vi "bbauv_acoustic_sbRIO_v3.vi"() -> ()   [LabVIEW 2012]
doc: "This VI will initialize the FPGA VI and read a user-defined number of samples from a DMA FIFO. When the data acquisition is complete this VI will read status information from the FPGA VI.\n\nFollow these instructions to run the VI.\n\n1. Select your RIO device from the dropdown.\n2. Set the sample period, number of samples to acquire per channel, and DMA block read size. \n\nNote: the block read size should be set to balance load on the host processor and the update rate of the user interface. A small block read size will update the user interface more often but will result in a higher load on the host processor."
uses:
  <vilib>/userdefined/High Color/nirio_resource_hc.ctl
  <vilib>/Analysis/3filter.llb/Filter Passband Type.ctl
  <vilib>/FPGAPlugInAG/sbRIO-9612/niLvFpga_Open_sbRIO-9612.vi
  <vilib>/rvi/interface/common/dynamic/niFpgaDynamicAddResources.vi
  <vilib>/Utility/error.llb/Error Cluster From Error Code.vi
  <vilib>/FPGAPlugInAG/Dynamic/niLvFpga_Run_Dynamic.vi
  <vilib>/rvi/errors/niLvFpgaAdjustHostInterfaceError.vi
  <vilib>/RVI Host/nirviSupport.llb/nirviErrorClusterFromErrorCode.vi
  <vilib>/FPGAPlugInAG/Dynamic/niLvFpga_Close_Dynamic.vi
  <vilib>/Analysis/3filter.llb/Elliptic Filter (DBL).vi
  <vilib>/Analysis/3filter.llb/Butterworth Filter (DBL).vi
  <vilib>/rvi/interface/nirviOpenFPGA/nirviOpenFPGA.xnode
  FPGA Bitfiles/bbauvFPGA_FPGATarget2_NI9223User-Contr_AXBjtBmtN8Y.lvbitx
  NI 9223 User-Controlled IO Sampling (FPGA).vi
  <vilib>/rvi/interface/nirviMethod/nirviMethod.xnode
  <vilib>/rvi/interface/nirviReadWriteControl/nirviReadWriteControl.xnode
  <vilib>/rvi/interface/nirviCloseFPGA/nirviCloseFPGA.xnode
  <vilib>/rvi/errors/niLvFpgaMergeErrorWithErrorCode.vi
  <vilib>/rvi/interface/Simulation/niFpgaSimulationCallBeginRW.vi
  <vilib>/FPGAPlugInAG/Dynamic/niLvFpga_ReadFifo_Dynamic.vi
  <vilib>/rvi/interface/nirviMethod/StockFPGA_InlinedMethodWaitForSingleIRQ.vi
  <vilib>/FPGAPlugInAG/Dynamic/niLvFpga_WaitOnIrq_Dynamic.vi
  <vilib>/FPGAPlugInAG/Dynamic/niLvFpga_AcknowledgeIrq_Dynamic.vi
  NiFpgaLv.dll
  <vilib>/FPGAPlugInAG/Dynamic/niLvFpga_ConfigureFifo_Dynamic.vi
  <vilib>/FPGAPlugInAG/Dynamic/niLvFpga_StartFifo_Dynamic.vi
  <vilib>/Analysis/NI_AALBase.lvlib
panel:
  out "Frequency":dbl
  in  "Noise length":i32=300
  out "Index 0":dbl
  out "Index 1":dbl
  out "Index 2":dbl
  out "Index 3":dbl
  out "amplitude 0":dbl
  out "amplitude 1":dbl
  out "amplitude 2":dbl
  out "amplitude 3":dbl
  in  "Portion Duration":i32=1000
  out "Threshold 0":dbl
  out "Threshold 1":dbl
  out "Threshold 2":dbl
  out "Threshold 3":dbl
  in  "threshold ratio":dbl=3.0
  in  "Display":bool
  in  "Filter mode":enum16{"Elliptic", "Butterworth"}(ring)=enum."Butterworth"
  out "Selected Index":i32
  out "Ratio at Index (%)":dbl
  in  "Threshold":dbl=0.3
  in  "Order":i32=3
  in  "Low Cutoff":dbl=20000.0
  in  "High Cutoff":dbl=26000.0
  in  "Selection:":dbl=25000.0
  out "Freq 2":dbl
  out "Freq 1":dbl
  out "Original Filtered Ch0":dbl[](graph)
  out "bad signal?":bool
  out "dt1":dbl
  out "dt2":dbl
  out "dt3":dbl
  out "ROS  Error":bool
  in  "Send to ROS":bool=TRUE
  in  "Altitude":dbl=2.0
  out "x":dbl format="%#_6f"
  out "y":dbl format="%#_6f"
  out "z":dbl
  out "yaw":dbl
  out "pitch":dbl
  in  "Mode":T1(ring)=enum."Use Far Field"
  out "Forward":dbl
  out "Sidemove":dbl
  out "Arrival Analysis Signal":dbl[][](graph)
  out "Yaw Chart":dbl(graph)
  out "noise index":dbl[](array[numeric])
  out "Frequency Selected Signal":dbl[](graph)
  out "#Elements Acquired":u32(graph)
  in  "Sampling Duration (us)":u32=2005000
  in  "RIO Device":T2="RIO0"
  out "Timed Out":bool
  out "Sample Gated":bool
  out "Overwrite":bool
  in  "Acquisition Stop":bool
  # "Signal Acquisition Control"
  # "TDOA Analysis"
  # "Arrival Analysis"
  # "Frequency Analysis"
  # "TDOA Result"
  # "ROS Communication"
  # "Frequency Analysis"
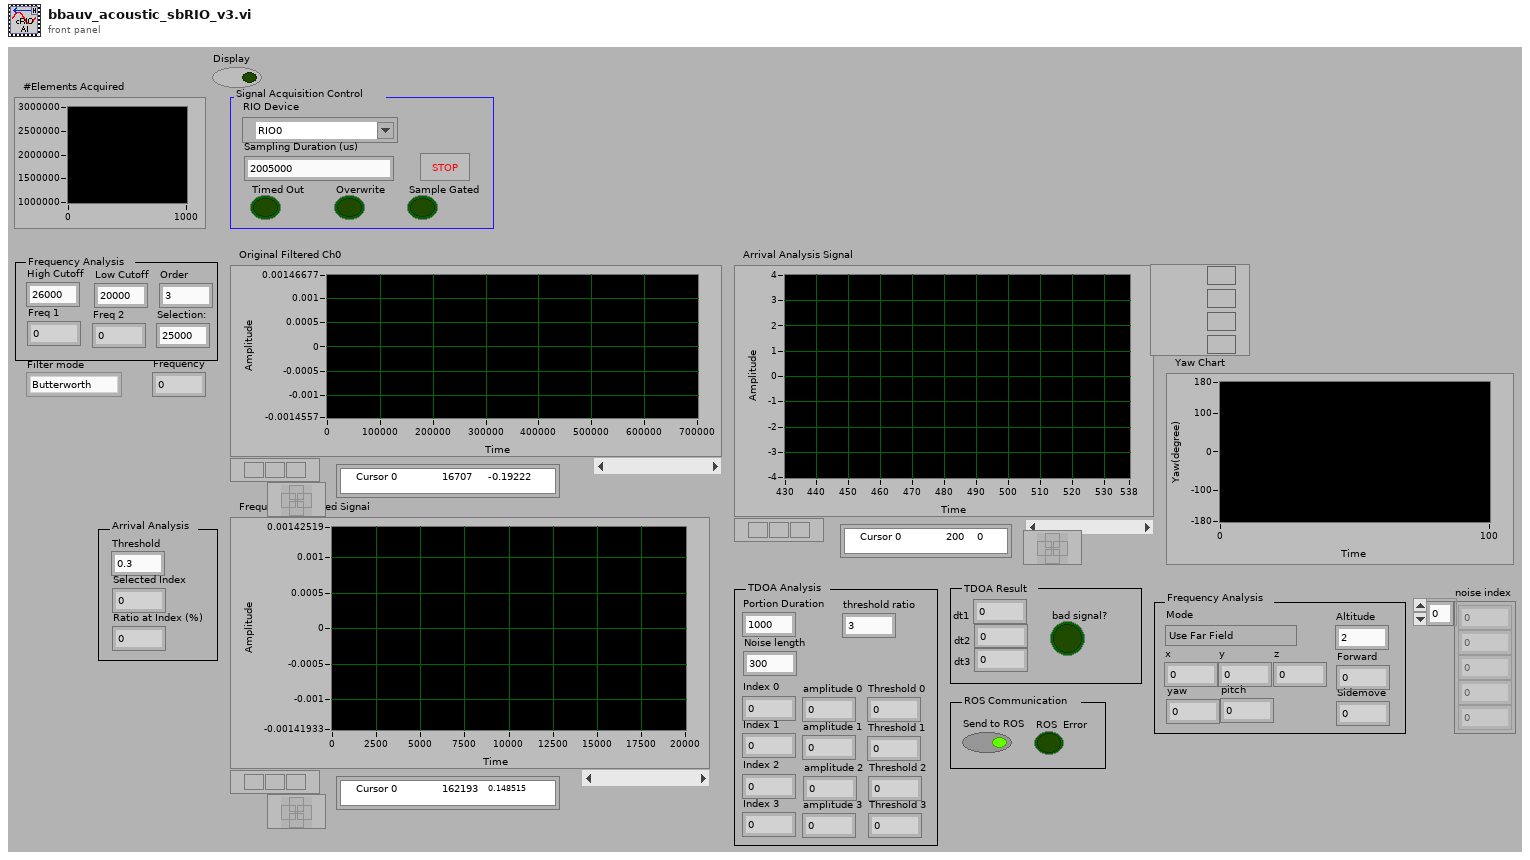
[diagram p1: front panel]
types:
  T1 = enum16{"Use Near Field", "Use Far Field", "Far Field with 3 hydrophones"}
  T2 = typedef "nirio_resource_hc.ctl" = tag
  T3 = typedef "NI_AALBase.lvlib/Filter Passband Type.ctl" = enum32{"Lowpass", "Highpass", "Bandpass", "Bandstop"}
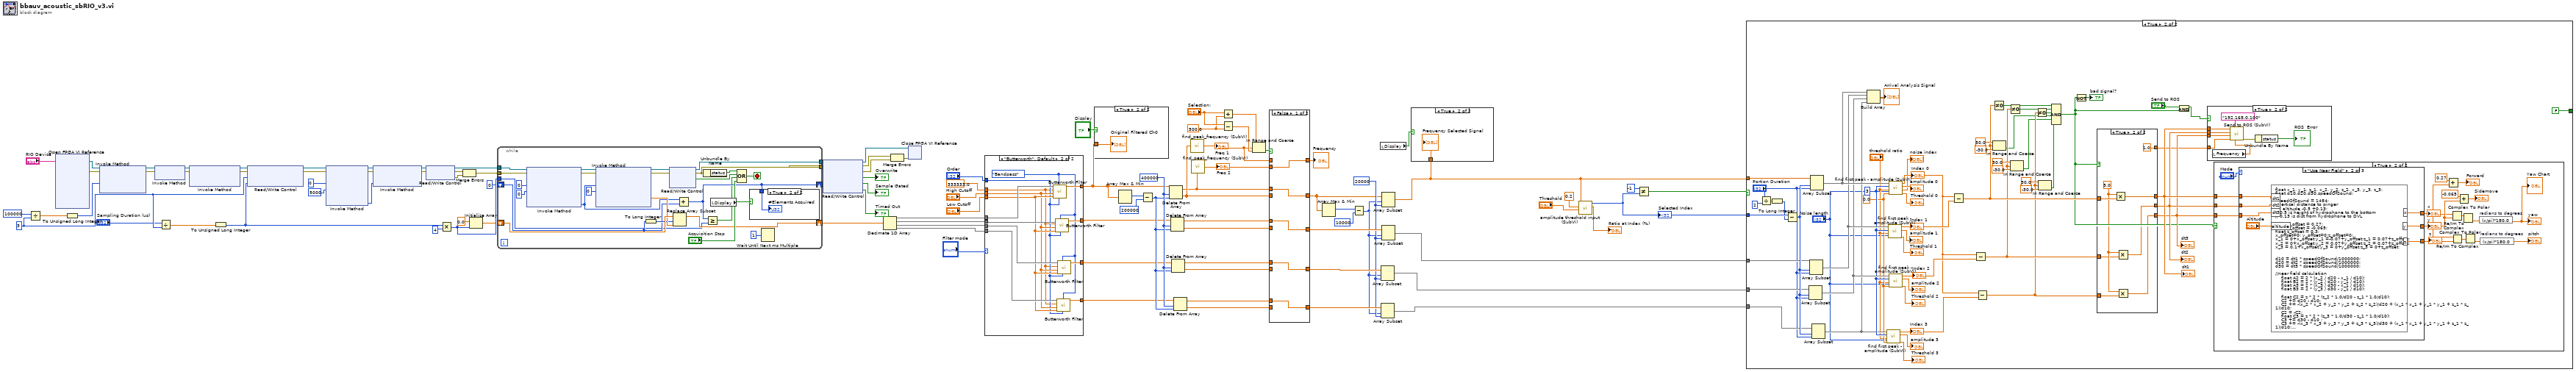
[diagram p0: block diagram]
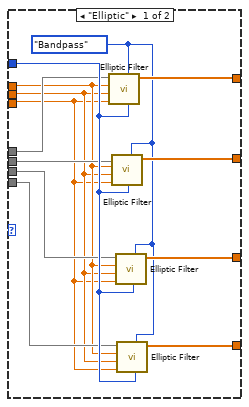
[diagram p4: hidden frame]
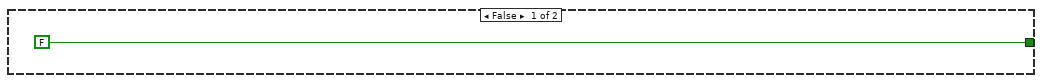
[diagram p5: hidden frame]
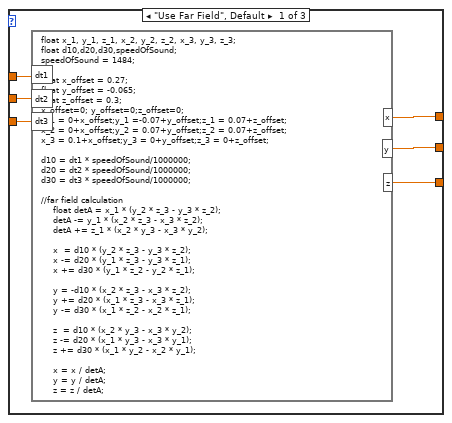
[diagram p7: hidden frame]
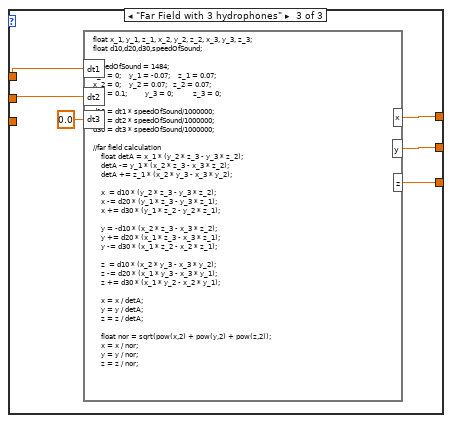
[diagram p8: hidden frame]
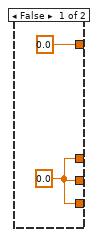
[diagram p10: hidden frame]
diagram:
  w33 = 500.0 ("y")
  w38 = 20000 ("length")
  w51 = 400000 ("Portion Duration")
  w58 = u32 3 ("Sample Period (uSec)")
  n1 = Divide(x=u32 100000, y=w58) -> (x/y=w91:dbl)
  n2 = xnode "Open FPGA VI Reference"("resource name"="RIO Device") -> ("FPGA VI Reference Out"=w94:refnum<k20>, "error out"=w93:errorcluster)  [unwired: 1 in]
  n3 = To Unsigned Long Integer(number=w91) -> (unsigned 32bit integer=w92:u32)
  n4 = xnode "Invoke Method"("FPGA VI Reference In"=w94, "error in"=w93, "Requested Depth"=w92) -> ("FPGA VI Reference Out"=w96:refnum<k20>, "error out"=w95:errorcluster)  [unwired: 1 out]
  n5 = xnode "Invoke Method"("FPGA VI Reference In"=w96, "error in"=w95) -> ("FPGA VI Reference Out"=w85:refnum<k20>, "error out"=w84:errorcluster)
  n6 = Divide(x="Sampling Duration (us)", y=w58) -> (x/y=w56:dbl)
  n7 = xnode "Invoke Method"("FPGA VI Reference In"=w85, "error in"=w84) -> ("FPGA VI Reference Out"=w61:refnum<k20>, "error out"=w60:errorcluster)  [unwired: 1 in]
  n8 = To Unsigned Long Integer(number=w56) -> (unsigned 32bit integer=w54:u32)
  n9 = xnode "Read/Write Control"("FPGA VI Reference In"=w61, "error in"=w60, "Sample Period (uSec)"=w58, "Number of Samples"=w54) -> ("FPGA VI Reference Out"=w75:refnum<k20>, "error out"=w74:errorcluster)
  n10 = xnode "Invoke Method"("FPGA VI Reference In"=w75, "error in"=w74, "IRQ Number(s)"=0, "Timeout (ms)"=5000) -> ("FPGA VI Reference Out"=w72:refnum<k20>, "error out"=w73:errorcluster, "IRQ(s) Asserted"=w69:i32)  [unwired: 1 out]
  n11 = xnode "Invoke Method"("FPGA VI Reference In"=w72, "error in"=w73, "IRQ Number(s)"=w69) -> ("FPGA VI Reference Out"=w71:refnum<k20>, "error out"=w70:errorcluster)
  n12 = xnode "Read/Write Control"("FPGA VI Reference In"=w71, "error in"=w70) -> ("FPGA VI Reference Out"=w63:refnum<k20>, "error out"=w77:errorcluster, "Error Out"=w76:errorcluster)
  n13 = Multiply(x=w54, y=u32 4) -> (x*y=w88:u32)
  n14 = Merge Errors(w77, w76) -> (w62:errorcluster)
  n15 = Initialize Array(sgl 0.0, w88) -> (w64:sgl[])
  n16 = while {
    tunnel: w63 -> [w110]
    tunnel: w62 -> [w109]
    tunnel: [w118] -> w83
    tunnel: [w117] -> w82
    shift-right: [w100] -> _
    shift-left: u32 0 -> [w111]
    tunnel: w88 -> [w103]
    shift-right: [w113] -> w55
    shift-left: w64 -> [w119]
    stop <- w120 stop-if-true
    n17 = xnode "Invoke Method"("FPGA VI Reference In"=w110, "error in"=w109, "Number of Elements"=u32 0, "Timeout (ms)"=0) -> ("FPGA VI Reference Out"=w108:refnum<k20>, "error out"=w107:errorcluster, "Elements Remaining"=w101:u32)  [unwired: 1 out]
    n18 = xnode "Invoke Method"("FPGA VI Reference In"=w108, "error in"=w107, "Number of Elements"=w101, "Timeout (ms)"=0) -> ("FPGA VI Reference Out"=w123:refnum<k20>, "error out"=w122:errorcluster, "Data"=w114:sgl[])  [unwired: 1 out]
    n19 = To Long Integer(number=w111) -> (32bit integer=w112:i32)
    n20 = xnode "Read/Write Control"("FPGA VI Reference In"=w123, "error in"=w122) -> ("FPGA VI Reference Out"=w118:refnum<k20>, "error out"=w117:errorcluster, "Error"=w102:bool)  [unwired: 1 out]
    n21 = Replace Array Subset(array=w119, new element=w114, index=w112) -> (w113:sgl[])
    n22 = Add(x=w101, y=w111) -> (x+y=w100:u32)
    n23 = Unbundle By Name(w117) -> ("status"=w104:bool)
    n24 = Greater Or Equal?(x=w100, y=w103) -> (x >= y?=w99:bool)
    n25 = local read "Display"() -> (w98:bool)
    n26 = Compound Arithmetic op=OR(w104, w102, w99, "Acquisition Stop") -> (w120:bool)
    n27 = case shown="True" w98 {
      tunnel: w100 -> [_ w124]
      frame False {
      }
      frame True {
        "#Elements Acquired" <- w124
      }
    }
    n28 = Wait Until Next ms Multiple(millisecond multiple=u32 1) -> ()  [unwired: 1 out]
  }
  n29 = xnode "Read/Write Control"("FPGA VI Reference In"=w83, "error in"=w82) -> ("FPGA VI Reference Out"=w87:refnum<k20>, "error out"=w78:errorcluster, "Error Out"=w79:errorcluster, "Overwrite"=→"Overwrite":bool, "Sample Gated"=→"Sample Gated":bool, "Timed Out"=→"Timed Out":bool)
  n30 = Decimate 1D Array(w55) -> (w4:sgl[], w14:sgl[], w15:sgl[], w13:sgl[])
  n31 = Merge Errors(w78, w79) -> (w86:errorcluster)
  n32 = xnode "Close FPGA VI Reference"("FPGA VI Reference In"=w87, "error in"=w86) -> ()  [unwired: 1 out]
  n33 = case shown="\"Butterworth\", Default" "Filter mode" {
    tunnel: w14 -> [w131 w150]
    tunnel: w13 -> [w129 w149]
    tunnel: w15 -> [w130 w148]
    tunnel: w4 -> [w132 w147]
    tunnel: [w137 w146] -> w5
    tunnel: [w136 w145] -> w8
    tunnel: [w135 w144] -> w7
    tunnel: [w134 w143] -> w6
    tunnel: "Low Cutoff" -> [w125 w142]
    tunnel: "High Cutoff" -> [w126 w141]
    tunnel: "Order" -> [w133 w140]
    tunnel: 333333.0 ("sampling freq: fs") -> [w127 w139]
    frame "Elliptic" {
      w128 = Filter_Passband_Type."Bandpass" ("filter type")
      n34 = call-poly <vilib>:"Elliptic Filter.vi"("order"=w133, "filter type"=w128, "low cutoff freq: fl"=w125, "high cutoff freq: fh"=w126, "sampling freq: fs"=w127, "X"=w132) -> ("Filtered X"=w137:dbl[])  [unwired: 4 in, 1 out]
      n35 = call-poly <vilib>:"Elliptic Filter.vi"("order"=w133, "filter type"=w128, "low cutoff freq: fl"=w125, "high cutoff freq: fh"=w126, "sampling freq: fs"=w127, "X"=w131) -> ("Filtered X"=w136:dbl[])  [unwired: 4 in, 1 out]
      n36 = call-poly <vilib>:"Elliptic Filter.vi"("order"=w133, "filter type"=w128, "low cutoff freq: fl"=w125, "high cutoff freq: fh"=w126, "sampling freq: fs"=w127, "X"=w130) -> ("Filtered X"=w135:dbl[])  [unwired: 4 in, 1 out]
      n37 = call-poly <vilib>:"Elliptic Filter.vi"("order"=w133, "filter type"=w128, "low cutoff freq: fl"=w125, "high cutoff freq: fh"=w126, "sampling freq: fs"=w127, "X"=w129) -> ("Filtered X"=w134:dbl[])  [unwired: 4 in, 1 out]
    }
    frame "Butterworth", Default {
      w138 = Filter_Passband_Type."Bandpass" ("filter type")
      n38 = call-poly <vilib>:"Butterworth Filter.vi"("order"=w140, "filter type"=w138, "low cutoff freq: fl"=w142, "high cutoff freq: fh"=w141, "sampling freq: fs"=w139, "X"=w147) -> ("Filtered X"=w146:dbl[])  [unwired: 2 in, 1 out]
      n39 = call-poly <vilib>:"Butterworth Filter.vi"("order"=w140, "filter type"=w138, "low cutoff freq: fl"=w142, "high cutoff freq: fh"=w141, "sampling freq: fs"=w139, "X"=w150) -> ("Filtered X"=w145:dbl[])  [unwired: 2 in, 1 out]
      n40 = call-poly <vilib>:"Butterworth Filter.vi"("order"=w140, "filter type"=w138, "low cutoff freq: fl"=w142, "high cutoff freq: fh"=w141, "sampling freq: fs"=w139, "X"=w149) -> ("Filtered X"=w143:dbl[])  [unwired: 2 in, 1 out]
      n41 = call-poly <vilib>:"Butterworth Filter.vi"("order"=w140, "filter type"=w138, "low cutoff freq: fl"=w142, "high cutoff freq: fh"=w141, "sampling freq: fs"=w139, "X"=w148) -> ("Filtered X"=w144:dbl[])  [unwired: 2 in, 1 out]
    }
  }
  n42 = case shown="True" "Display" {
    tunnel: w5 -> [_ w151]
    frame False {
    }
    frame True {
      "Original Filtered Ch0" <- w151
    }
  }
  n43 = Array Max & Min(array=w5) -> (max index (indices)=w53:i32)  [unwired: 3 out]
  n44 = Subtract(x=w53, y=200000) -> (x-y=w50:i32)
  n45 = Delete From Array(array=w5, length=w51, index=w50) -> (deleted portion=w36:dbl[], array with subset deleted=w35:dbl[])
  n46 = Delete From Array(array=w8, length=w51, index=w50) -> (deleted portion=w49:dbl[], array with subset deleted=w46:dbl[])
  n47 = Delete From Array(array=w7, length=w51, index=w50) -> (deleted portion=w48:dbl[], array with subset deleted=w45:dbl[])
  n48 = Delete From Array(array=w6, length=w51, index=w50) -> (deleted portion=w47:dbl[], array with subset deleted=w44:dbl[])
  n49 = call "find_peak_frequency (SubVI).vi"("Signal"=w36) -> ("Frequency"=w29:dbl)
  "Freq 1" <- w29
  n50 = call "find_peak_frequency (SubVI).vi"("Signal"=w35) -> ("Frequency"=w28:dbl)
  "Freq 2" <- w28
  n51 = Add(x="Selection:", y=w33) -> (x+y=w31:dbl)
  n52 = Subtract(x="Selection:", y=w33) -> (x-y=w30:dbl)
  n53 = In Range and Coerce(upper limit=w31, x=w29, lower limit=w30) -> (In Range?=w32:bool)  [unwired: 1 out]
  n54 = case shown="False" w32 {
    tunnel: w36 -> [_ w161]
    tunnel: w49 -> [_ w160]
    tunnel: w48 -> [_ w159]
    tunnel: w47 -> [_ w158]
    tunnel: w35 -> [w156 _]
    tunnel: w46 -> [w155 _]
    tunnel: w45 -> [w154 _]
    tunnel: w44 -> [w153 _]
    tunnel: [w156 w161] -> w17
    tunnel: [w155 w160] -> w41
    tunnel: [w154 w159] -> w40
    tunnel: [w153 w158] -> w39
    tunnel: [w152 w157] -> w1
    tunnel: w29 -> [_ w157]
    tunnel: w28 -> [w152 _]
    frame False {
    }
    frame True {
    }
  }
  "Frequency" <- w1
  n55 = Array Max & Min(array=w17) -> (max index (indices)=w42:i32)  [unwired: 3 out]
  n56 = Subtract(x=w42, y=10000) -> (x-y=w37:i32)
  n57 = local read "Display"() -> (w2:bool)
  n58 = Array Subset(array=w40, index=w37, length=w38) -> (w25:dbl[])
  n59 = Array Subset(array=w39, index=w37, length=w38) -> (w24:dbl[])
  n60 = Array Subset(array=w17, index=w37, length=w38) -> (w21:dbl[])
  n61 = Array Subset(array=w41, index=w37, length=w38) -> (w26:dbl[])
  n62 = case shown="True" w2 {
    tunnel: w21 -> [_ w162]
    frame False {
    }
    frame True {
      "Frequency Selected Signal" <- w162
    }
  }
  n63 = call "amplitude threshold input (SubVI).vi"("threshold"="Threshold", "%max amplitude"=0.2, "Array"=w21) -> ("actual ratio (%)"=→"Ratio at Index (%)":dbl, "Index"=w18:i32)  [unwired: 7 in]
  "Selected Index" <- w18
  n64 = Not Equal?(x=-1 ("y"), y=w18) -> (x != y?=w23:bool)
  n65 = case shown="True" w23 {
    tunnel: w26 -> [_ w218]
    tunnel: w25 -> [_ w217]
    tunnel: w24 -> [_ w216]
    tunnel: w21 -> [_ w215]
    tunnel: w18 -> [_ w214]
    tunnel: [FALSE ("Debug") FALSE ("Debug")] -> _
    frame False {
    }
    frame True {
      w183 = 0.0 ("noise min")
      w188 = 3
      n66 = Divide(x="Portion Duration", y=2) -> (x/y=w211:dbl)
      n67 = To Long Integer(number=w211) -> (32bit integer=w210:i32)
      n68 = Subtract(x=w214, y=w210) -> (x-y=w219:i32)
      n69 = Array Subset(array=w217, index=w219, length="Portion Duration") -> (w189:dbl[])
      n70 = Array Subset(array=w218, index=w219, length="Portion Duration") -> (w193:dbl[])
      n71 = Array Subset(array=w215, index=w219, length="Portion Duration") -> (w195:dbl[])
      n72 = Array Subset(array=w216, index=w219, length="Portion Duration") -> (w187:dbl[])
      n73 = Build Array(w195, w193, w189, w187) -> (→"Arrival Analysis Signal":dbl[][])
      n74 = call "find first peak - amplitude (SubVI).vi"("Noise duration (units)"="Noise length", "Noise min (amplitude)"=w183, "threshold ratio"="threshold ratio", "peak width (units)"=w188, "Array"=w187) -> ("Peak threshold"=→"Threshold 3":dbl, "peak amplitude"=→"amplitude 3":dbl, "Index"=w186:dbl)  [unwired: 2 in, 2 out]
      "Index 3" <- w186
      n75 = call "find first peak - amplitude (SubVI).vi"("Noise duration (units)"="Noise length", "threshold ratio"="threshold ratio", "peak width (units)"=w188, "Array"=w193) -> ("Peak threshold"=→"Threshold 1":dbl, "peak amplitude"=→"amplitude 1":dbl, "Index"=w192:dbl)  [unwired: 3 in, 2 out]
      "Index 1" <- w192
      n76 = call "find first peak - amplitude (SubVI).vi"("Noise duration (units)"="Noise length", "Noise min (amplitude)"=w183, "threshold ratio"="threshold ratio", "peak width (units)"=w188, "Array"=w195) -> ("Peak threshold"=→"Threshold 0":dbl, "noise index"=→"noise index":dbl[], "peak amplitude"=→"amplitude 0":dbl, "Index"=w182:dbl)  [unwired: 2 in, 1 out]
      "Index 0" <- w182
      n77 = call "find first peak - amplitude (SubVI).vi"("Noise duration (units)"="Noise length", "Noise min (amplitude)"=w183, "threshold ratio"="threshold ratio", "peak width (units)"=w188, "Array"=w189) -> ("Peak threshold"=→"Threshold 2":dbl, "peak amplitude"=→"amplitude 2":dbl, "Index"=w190:dbl)  [unwired: 2 in, 2 out]
      "Index 2" <- w190
      n78 = Subtract(x=w182, y=w192) -> (x-y=w173:dbl)
      n79 = Subtract(x=w182, y=w190) -> (x-y=w172:dbl)
      n80 = Subtract(x=w182, y=w186) -> (x-y=w171:dbl)
      n81 = Not Equal To 0?(x=w173) -> (x != 0?=w170:bool)
      n82 = In Range and Coerce(upper limit=30.0, x=w173, lower limit=-30.0) -> (In Range?=w167:bool)  [unwired: 1 out]
      n83 = Not Equal To 0?(x=w172) -> (x != 0?=w169:bool)
      n84 = In Range and Coerce(upper limit=30.0, x=w172, lower limit=-30.0) -> (In Range?=w166:bool)  [unwired: 1 out]
      n85 = Not Equal To 0?(x=w171) -> (x != 0?=w168:bool)
      n86 = In Range and Coerce(upper limit=30.0, x=w171, lower limit=-30.0) -> (In Range?=w165:bool)  [unwired: 1 out]
      n87 = Compound Arithmetic op=AND(w170, w169, w168, w167, w166, w165) -> (w164:bool)
      n88 = Not(x=w164) -> (.not. x?=→"bad signal?":bool)
      n89 = case shown="True" w164 {
        tunnel: w173 -> [_ w273]
        tunnel: w172 -> [_ w271]
        tunnel: w171 -> [_ w270]
        tunnel: [w264 w269] -> w200
        tunnel: [w264 w268] -> w199
        tunnel: [w264 w267] -> w198
        tunnel: [0.0 ("x") 1.0 ("x")] -> w197
        frame False {
          w264 = 0.0
        }
        frame True {
          w272 = 3.0 ("x")
          n90 = Multiply(x=w272, y=w273) -> (x*y=w269:dbl)
          n91 = Multiply(x=w272, y=w271) -> (x*y=w268:dbl)
          n92 = Multiply(x=w272, y=w270) -> (x*y=w267:dbl)
        }
      }
      "dt1" <- w200
      "dt2" <- w199
      "dt3" <- w198
      n93 = And(x="Send to ROS", y=w164) -> (x .and. y?=w196:bool)
      n94 = case shown="True" w196 {
        tunnel: w200 -> [_ w260]
        tunnel: w199 -> [_ w259]
        tunnel: w198 -> [_ w258]
        tunnel: w197 -> [_ w257]
        frame False {
        }
        frame True {
          n95 = local read "Frequency"() -> (w256:dbl)
          n96 = call "Send to ROS (SubVI).vi"("frequency"=w256, "ROS IP"="192.168.0.100", "Good signal?"=w257, "dt 3"=w258, "dt2"=w259, "dt 1"=w260) -> ("error out"=w262:errorcluster)  [unwired: 5 in]
          n97 = Unbundle By Name(w262) -> ("status"=→"ROS  Error":bool)
        }
      }
      n98 = case shown="True" w164 {
        tunnel: w200 -> [_ w228]
        tunnel: w199 -> [_ w227]
        tunnel: w198 -> [_ w226]
        frame False {
        }
        frame True {
          n99 = case shown="\"Use Near Field\"" "Mode" {
            tunnel: [w242 w249 w254] -> w220
            tunnel: [w241 w248 w253] -> w223
            tunnel: [w240 w247 w252] -> w232
            tunnel: w228 -> [w239 w245 w251]
            tunnel: w227 -> [w238 w244 w250]
            tunnel: w226 -> [w237 w243 _]
            frame "Use Far Field", Default {
              n100 = formula code="float x_1, y_1, z_1, x_2, y_2, z_2, x_3, y_3, z_3;\nfloat d10,d20,d30,speedOfSound;\nspeedOfSound = 1484;\n\nfloat x_offset = 0.27;\nfloat y_offset = -0.065;\nfloat z_offset = 0.3;\nx_offset=0; y_offset=0;z_offset=0;\nx_1 = 0+x_offset;y_1 =-0.07+y_offset;z_1 = 0.07+z_offset;\nx_2 = 0+x_offset;y_2 = 0.07+y_offset;z_2 = 0.07+z_offset;\nx_3 = 0.1+x_offset;y_3 = 0+y_offset;z_3 = 0+z_offset;\n\nd10 = dt1 * speedOfSound/1000000;\nd20 = dt2 * speedOfSound/1000000;\nd30 = dt3 * speedOfSound/1000000;\n\n//far field calculation\n    float detA = x_1 * (y_2 * z_3 - y_3 * z_2);\n    detA -= y_1 * (x_2 * z_3 - x_3 * z_2);\n    detA += z_1 * (x_2 * y_3 - x_3 * y_2);\n\n    x  = d10 * (y_2 * z_3 - y_3 * z_2);\n    x -= d20 * (y_1 * z_3 - y_3 * z_1);\n    x += d30 * (y_1 * z_2 - y_2 * z_1);\n\n    y = -d10 * (x_2 * z_3 - x_3 * z_2);\n    y += d20 * (x_1 * z_3 - x_3 * z_1);\n    y -= d30 * (x_1 * z_2 - x_2 * z_1);\n\n    z  = d10 * (x_2 * y_3 - x_3 * y_2);\n    z -= d20 * (x_1 * y_3 - x_3 * y_1);\n    z += d30 * (x_1 * y_2 - x_2 * y_1);\n\n    x = x / detA;\n    y = y / detA;\n    z = z / detA;\n\n    float nor = sqrt(pow(x,2) + pow(y,2) + pow(z,2));\n    x = x / nor;\n    y = y / nor;\n    z = z / nor;"("dt1"=w239, "dt2"=w238, "dt3"=w237) -> ("x"=w242:dbl, "y"=w241:dbl, "z"=w240:dbl)
            }
            frame "Use Near Field" {
              n101 = formula code="float x_1, y_1, z_1, x_2, y_2, z_2, x_3, y_3, z_3;\nfloat d10,d20,d30,speedOfSound;\n\nspeedOfSound = 1484;\n//vertical distance to pinger\nz= altitude -0.5 +0.13;\n// 0.5 is height of hydrophone to the bottom\n// 0.13 is dist from hydrophone to DVL\n\nfloat x_offset = 0.27;\nfloat y_offset = -0.065;\nfloat z_offset = 0.3;\nx_offset=0; y_offset=0;z_offset=0;\nx_1 = 0+x_offset;y_1 =-0.07+y_offset;z_1 = 0.07+z_offset;\nx_2 = 0+x_offset;y_2 = 0.07+y_offset;z_2 = 0.07+z_offset;\nx_3 = 0.1+x_offset;y_3 = 0+y_offset;z_3 = 0+z_offset;\n\n\nd10 = dt1 * speedOfSound/1000000;\nd20 = dt2 * speedOfSound/1000000;\nd30 = dt3 * speedOfSound/1000000;\n\n//near field calculation\n    float A2 = 2 * (x_2 / d20 - x_1 / d10);\n    float B2 = 2 * (y_2 / d20 - y_1 / d10);\n    float A3 = 2 * (x_3 / d30 - x_1 / d10);\n    float B3 = 2 * (y_3 / d30 - y_1 / d10);\n    \n    float C2 = z * 2 * (z_2 * 1.0/d20 - z_1 * 1.0/d10);\n    C2 += d20 - d10;\n    C2 += -(x_2 * x_2 + y_2 * y_2 + z_2 * z_2)/d20 + (x_1 * x_1 + y_1 * y_1 + z_1 * z_1)/d10;\n    C2 = -C2;\n    float C3 = z * 2 * (z_3 * 1.0/d30 - z_1 * 1.0/d10);\n    C3 += d30 - d10 ;\n    C3 += -(x_3 * x_3 + y_3 * y_3 + z_3 * z_3)/d30 + (x_1 * x_1 + y_1 * y_1 + z_1 * z_1)/d10;\n    C3 = -C3;\n\n    if (A2*B3 == A3*B2) {\n        x = 0;\n        y = 0;\n    }\n    else {\n        x = (C2 * B3 - C3 * B2) / (A2 * B3 - A3 * B2);\n        y = (C3 * A2 - C2 * A3) / (B3 * A2 - B2 * A3);\n    }"("dt1"=w245, "dt2"=w244, "dt3"=w243, "altitude"="Altitude") -> ("x"=w249:dbl, "y"=w248:dbl, "z"=w247:dbl)
            }
            frame "Far Field with 3 hydrophones" {
              n102 = formula code="float x_1, y_1, z_1, x_2, y_2, z_2, x_3, y_3, z_3;\nfloat d10,d20,d30,speedOfSound;\n\nspeedOfSound = 1484;\nx_1 = 0;    y_1 = -0.07;    z_1 = 0.07;\nx_2 = 0;    y_2 = 0.07;   z_2 = 0.07;\nx_3 = 0.1;         y_3 = 0;          z_3 = 0;\n\nd10 = dt1 * speedOfSound/1000000;\nd20 = dt2 * speedOfSound/1000000;\nd30 = dt3 * speedOfSound/1000000;\n\n//far field calculation\n    float detA = x_1 * (y_2 * z_3 - y_3 * z_2);\n    detA -= y_1 * (x_2 * z_3 - x_3 * z_2);\n    detA += z_1 * (x_2 * y_3 - x_3 * y_2);\n\n    x  = d10 * (y_2 * z_3 - y_3 * z_2);\n    x -= d20 * (y_1 * z_3 - y_3 * z_1);\n    x += d30 * (y_1 * z_2 - y_2 * z_1);\n\n    y = -d10 * (x_2 * z_3 - x_3 * z_2);\n    y += d20 * (x_1 * z_3 - x_3 * z_1);\n    y -= d30 * (x_1 * z_2 - x_2 * z_1);\n\n    z  = d10 * (x_2 * y_3 - x_3 * y_2);\n    z -= d20 * (x_1 * y_3 - x_3 * y_1);\n    z += d30 * (x_1 * y_2 - x_2 * y_1);\n\n    x = x / detA;\n    y = y / detA;\n    z = z / detA;\n\n    float nor = sqrt(pow(x,2) + pow(y,2) + pow(z,2));\n    x = x / nor;\n    y = y / nor;\n    z = z / nor;"("dt1"=w251, "dt2"=w250, "dt3"=0.0 ("input variable")) -> ("x"=w254:dbl, "y"=w253:dbl, "z"=w252:dbl)
            }
          }
          "x" <- w220
          "y" <- w223
          "z" <- w232
          n103 = Add(x=0.27, y=w220) -> (x+y=→"Forward":dbl)
          n104 = Re/Im To Complex(1:w223, 2:w220) -> (0:w230:cdb)
          n105 = Re/Im To Complex(1:w232, 2:w220) -> (0:w233:cdb)
          n106 = Add(x=-0.065, y=w223) -> (x+y=→"Sidemove":dbl)
          n107 = Complex To Polar(r * e^(i*theta)=w230) -> (theta=w231:dbl)  [unwired: 1 out]
          n108 = Complex To Polar(r * e^(i*theta)=w233) -> (theta=w235:dbl)  [unwired: 1 out]
          n109 = expression code="(x/pi)*180.0" "radians to degrees"(w231) -> (→"yaw" →"Yaw Chart":dbl)
          n110 = expression code="(x/pi)*180.0" "radians to degrees"(w235) -> (→"pitch":dbl)
        }
      }
    }
  }
